vi "Finalize View Init.vi"(8 "error in (no error)":errorcluster, 10 "View Name":string, 11 "Example Controller Actor in":refnum<class "Example Controller.lvclass">) -> (0 "error out":errorcluster, 3 "Example Controller Actor out":refnum<class "Example Controller.lvclass">)   [LabVIEW 2023, in "Example MVC Actors.lvlib" / "Example Controller.lvlib" / "Example Controller.lvclass"]
uses:
  Example Controller.lvclass
  Example Events/Inited At Event.lvclass
  Controller/Controller.lvclass/Controller.ctl
  Event Handlers/Abstract Event Message for View/Abstract Event Message for View.lvclass/Abstract Event Message for View.ctl
  <vilib>/ActorFramework/Message Enqueuer/Message Enqueuer.lvclass/Message Enqueuer.ctl
  Controller/Get View Details.vi
  Controller/Get Event Handlers Dict.vi
  Controller/Generate Event to View Core.vi
  Event Handlers/Abstract Event Message for View/Send Abstract Event Message for View.vi
  <vilib>/Utility/error.llb/Clear Errors.vi
  <vilib>/ActorFramework/Message Enqueuer/Enqueue.vi
  Event Handlers/Abstract Event Message for View/Abstract Event Message for View.lvclass
  <vilib>/Utility/error.llb/Error Cluster From Error Code.vi
  <vilib>/Utility/LVClass/Get LV Class Name.vi
  <resource>/AFDebug/Generate Trace for Message.vi
  <vilib>/ActorFramework/Message Priority Queue/Priority Enqueue.vi
  <vilib>/ErrorRing/Error Ring.xnode
  <vilib>/ActorFramework/Message Enqueuer/Message Enqueuer.lvclass
  Event/Event.lvclass
  Controller/Controller.lvclass
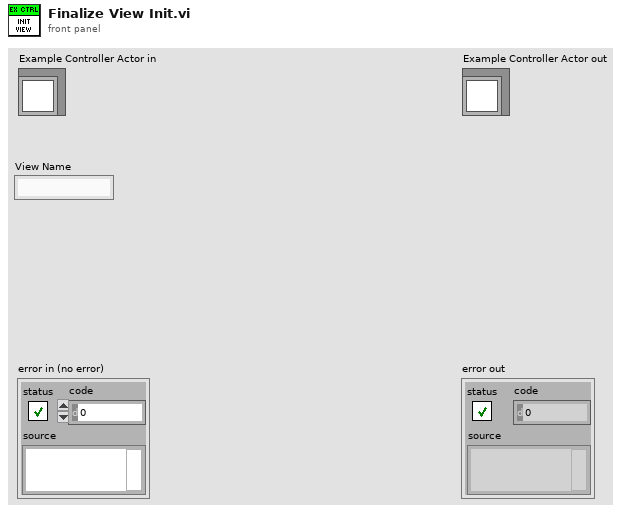
[diagram p1: front panel]
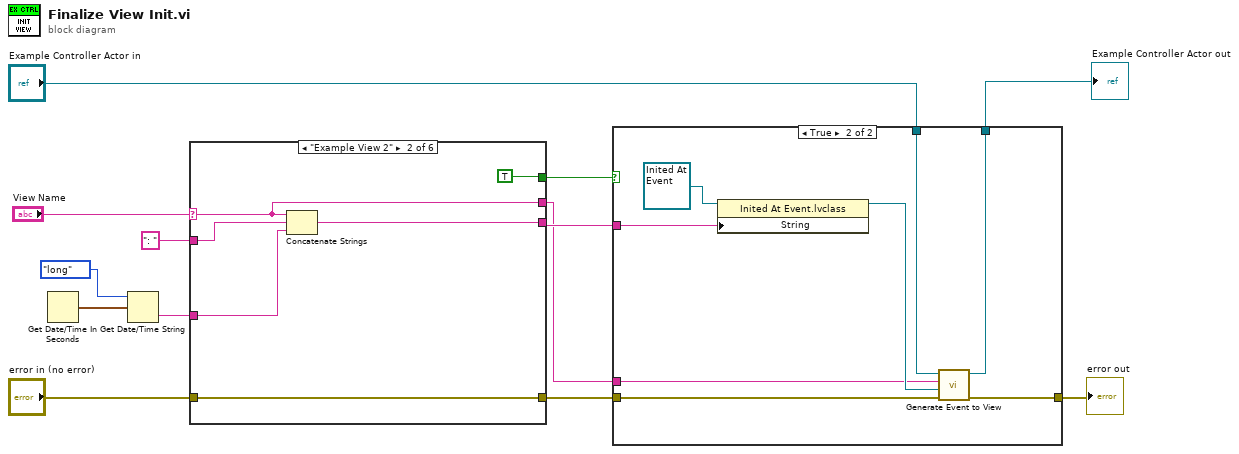
[diagram p0: block diagram]
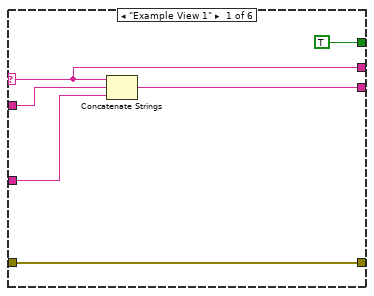
[diagram p3: hidden frame]
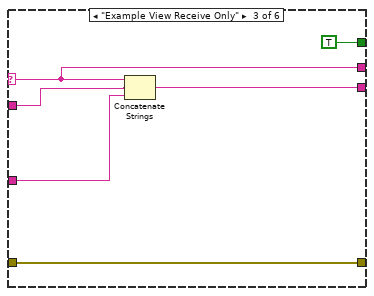
[diagram p4: hidden frame]
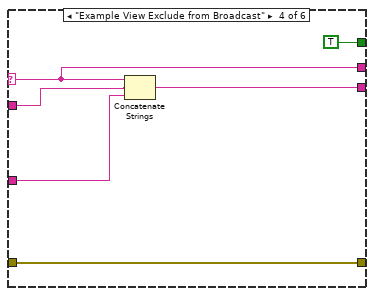
[diagram p5: hidden frame]
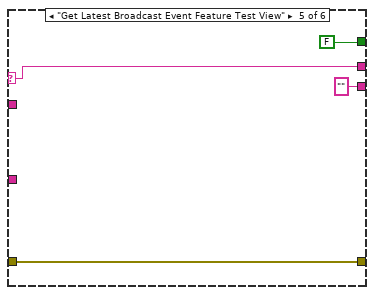
[diagram p6: hidden frame]
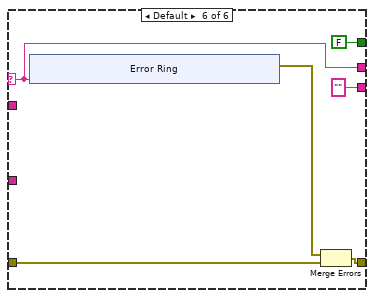
[diagram p7: hidden frame]
diagram:
  n1 = Get Date/Time In Seconds() -> (seconds since 1Jan1904=w12:timestamp)
  n2 = Get Date/Time String(date format (0)=enum16{"short", "long", "abbreviated"}."long", seconds (now)=w12) -> (time string=w10:string)  [unwired: 1 in, 1 out]
  n3 = case shown="\"Example View 2\"" "View Name" {
    selector: "View Name" -> [w16 w21 w28 w34 w41 w43]
    tunnel: w10 -> [w19 w25 w31 w37 _ _]
    tunnel: [w18 w23 w29 w35 "" ""] -> w5
    tunnel: "error in (no error)" -> [w15 w22 w27 w33 w39 w46]
    tunnel: [w15 w22 w27 w33 w39 w45] -> w7
    tunnel: ": " -> [w17 w24 w30 w36 _ _]
    tunnel: [w16 w21 w28 w34 w41 w43] -> w4
    tunnel: [TRUE TRUE TRUE TRUE FALSE FALSE] -> w1
    frame "Example View 1" {
      n4 = Concatenate Strings(w16, w17, w19) -> (w18:string)
    }
    frame "Example View 2" {
      n5 = Concatenate Strings(w21, w24, w25) -> (w23:string)
    }
    frame "Example View Receive Only" {
      n6 = Concatenate Strings(w28, w30, w31) -> (w29:string)
    }
    frame "Example View Exclude from Broadcast" {
      n7 = Concatenate Strings(w34, w36, w37) -> (w35:string)
    }
    frame "Get Latest Broadcast Event Feature Test View" {
    }
    frame Default {
      n8 = xnode "Error Ring"("parameter 0"=w43) -> ("error out"=w47:errorcluster)
      n9 = Merge Errors(w47, w46) -> (w45:errorcluster)
    }
  }
  n10 = case shown="True" w1 {
    tunnel: w7 -> [w55 w63]
    tunnel: [w55 w62] -> w6
    tunnel: w5 -> [_ w61]
    tunnel: w4 -> [_ w59]
    tunnel: "Example Controller Actor in" -> [w56 w58]
    tunnel: [w56 w57] -> w2
    frame False {
    }
    frame True {
      n11 = property class="Inited At Event.lvclass"(reference=refnum<class "Inited At Event.lvclass"> refnum ("Inited At Event.lvclass"), "String"=w61) -> (reference out=w60:refnum<class "Inited At Event.lvclass">)  [unwired: 1 in, 1 out]
      n12 = call "Generate Event to View.vi"("error in"=w63, "Event"=w60, "View Name"=w59, "Controller In"=w58) -> ("error out"=w62:errorcluster, "Controller Out"=w57:refnum<class "Example Controller.lvclass">)  [unwired: 6 in]
    }
  }
  "error out" <- w6
  "Example Controller Actor out" <- w2
